vi "Open Hardware.vi"(8 "error in (no error)":errorcluster, 11 "Inst.Krohn-Hite-7008 in":refnum<class "Inst.Krohn-Hite-7008.lvclass">) -> (0 "error out":errorcluster, 3 "Inst.Krohn-Hite-7008 out":refnum<class "Inst.Krohn-Hite-7008.lvclass">)   [LabVIEW 2019, in "Inst.KH7008.lvlib" / "Inst.Krohn-Hite-7008.lvclass"]
uses:
  Inst.Krohn-Hite-7008.lvclass
  C:/Program Files/National Instruments/LabVIEW 2019/user.lib/LevyLab/Instrument Framework/Instrument/Instrument.lvclass
  C:/Program Files/National Instruments/LabVIEW 2019/vi.lib/JKI/JKI SMO/SMO/SMO.lvclass
  <userlib>/LevyLab/Instrument Framework/Instrument/Instrument.lvclass/Instrument.ctl
  Inst.Krohn-Hite-7008.lvclass/Inst.Krohn-Hite-7008.ctl
  <userlib>/LevyLab/Instrument Framework/Instrument Types/Amplifier/Instrument.Amplifier.lvclass
  KH7008/KH7008.lvlib
  <vilib>/JKI/JKI SMO/SMO/SMO.lvclass
  <userlib>/LevyLab/Instrument Framework/Instrument/Instrument.lvclass
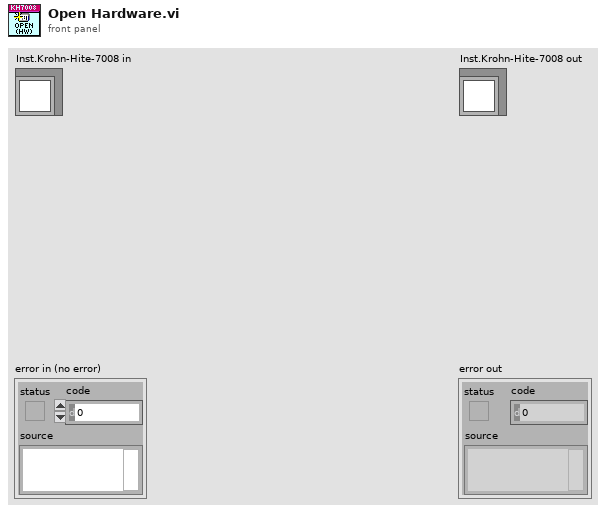
[diagram p1: front panel]
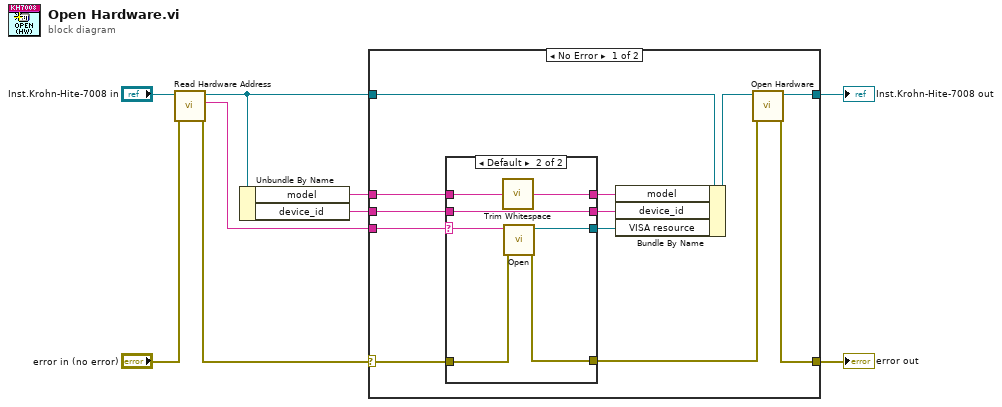
[diagram p0: block diagram]
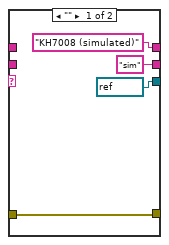
[diagram p2: hidden frame]
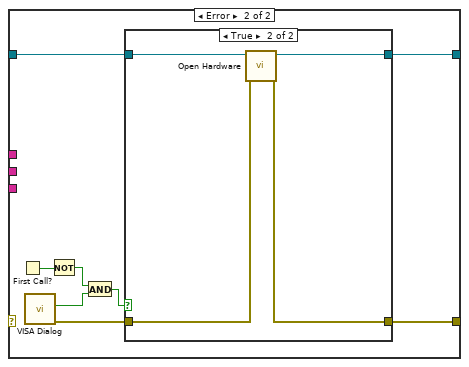
[diagram p3: hidden frame]
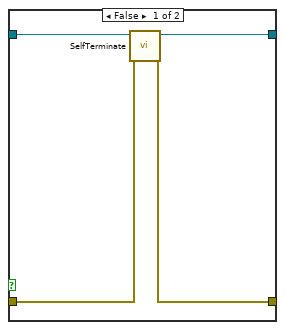
[diagram p4: hidden frame]
diagram:
  n1 = call <userlib>:"Read Hardware Address.vi"("error in (no error)"="error in (no error)", "Instrument in"="Inst.Krohn-Hite-7008 in") -> ("error out"=w2:errorcluster, "Address"=w1:string, "Instrument out"=w5:refnum<class "Inst.Krohn-Hite-7008.lvclass">)  [unwired: 7 in]
  n2 = Unbundle By Name(w5) -> ("model"=w7:string, "device_id"=w6:string)
  n3 = case shown="No Error" w2 {
    selector: w2 -> [w21 _]
    tunnel: [w15 w38] -> w9
    tunnel: w5 -> [w14 w39]
    tunnel: [w16 w40] -> w8
    tunnel: w7 -> [w13 _]
    tunnel: w6 -> [w12 _]
    tunnel: w1 -> [w11 _]
    frame No Error {
      n4 = case shown="Default" w11 {
        selector: w11 -> [_ w31]
        tunnel: w21 -> [w25 w29]
        tunnel: [w25 w28] -> w20
        tunnel: [refnum<visa-resource-name> "sim" ("VISA resource name out") w30] -> w19
        tunnel: w12 -> [_ w32]
        tunnel: ["sim" ("Serial Number") w32] -> w18
        tunnel: w13 -> [_ w26]
        tunnel: ["KH7008 (simulated)" ("Description") w27] -> w17
        frame "" {
        }
        frame Default {
          n5 = call <vilib>:"Trim Whitespace.vi"("string"=w26) -> ("trimmed string"=w27:string)  [unwired: 1 in]
          n6 = call "Open.vi"("error in (no error)"=w29, "VISA resource name"=w31) -> ("error out"=w28:errorcluster, "VISA resource"=w30:refnum<visa-resource-name>)  [unwired: 8 in]
        }
      }
      n7 = Bundle By Name(cluster=w14, "model"=w17, "device_id"=w18, "VISA resource"=w19) -> (w10:refnum<class "Inst.Krohn-Hite-7008.lvclass">)
      n8 = call-parent "Open Hardware.vi"("error in (no error)"=w20, "Instrument in"=w10) -> ("error out"=w15:errorcluster, "Instrument out"=w16:refnum<class "Inst.Krohn-Hite-7008.lvclass">)  [unwired: 8 in]
    }
    frame Error {
      n9 = First Call?() -> (First Call?: T/F=w36:bool)
      n10 = call "VISA Dialog.vi"() -> ("error out"=w37:errorcluster, "OK button"=w34:bool)  [unwired: 10 in]
      n11 = Not(x=w36) -> (.not. x?=w35:bool)
      n12 = And(x=w35, y=w34) -> (x .and. y?=w33:bool)
      n13 = case shown="True" w33 {
        tunnel: w39 -> [w42 w48]
        tunnel: [w43 w47] -> w40
        tunnel: w37 -> [w41 w46]
        tunnel: [w44 w45] -> w38
        frame False {
          n14 = call <vilib>:"SelfTerminate.vi"("error in (no error)"=w41, "SMO in"=w42) -> ("error out"=w44:errorcluster, "SMO out"=w43:refnum<class "Inst.Krohn-Hite-7008.lvclass">)  [unwired: 8 in]
        }
        frame True {
          n15 = call-dynamic "Open Hardware.vi"("error in (no error)"=w46, "Inst.Krohn-Hite-7008 in"=w48) -> ("error out"=w45:errorcluster, "Inst.Krohn-Hite-7008 out"=w47:refnum<class "Inst.Krohn-Hite-7008.lvclass">)  [unwired: 8 in]
        }
      }
    }
  }
  "error out" <- w9
  "Inst.Krohn-Hite-7008 out" <- w8
